vi "OP150ZP_SCANequipements.vi"(8 "Errin":errorcluster caption="errin", 10 "Chaîne":string="Log et conf\\Config.ini", 11 "pathin":path=path "D:/CODE/02 SLIM ZEN") -> (0 "ERROUT":errorcluster caption="error out", 1 "KO?":bool=TRUE)   [LabVIEW 2020]
doc: "Ce vi il détecte la presence des équipements"
uses:
  Documents/GitHub/ZEN-PLUS/OP150/EN PRODUCTION/OP150/VG/VG_BT3562.vi
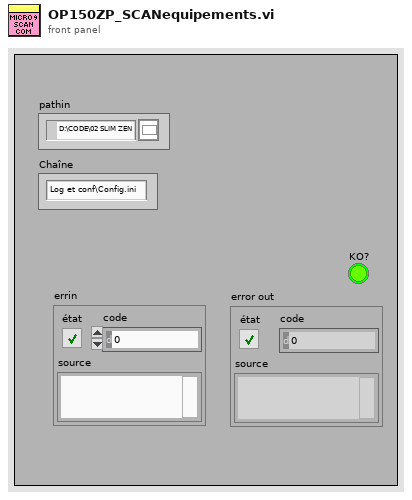
[diagram p1: front panel]
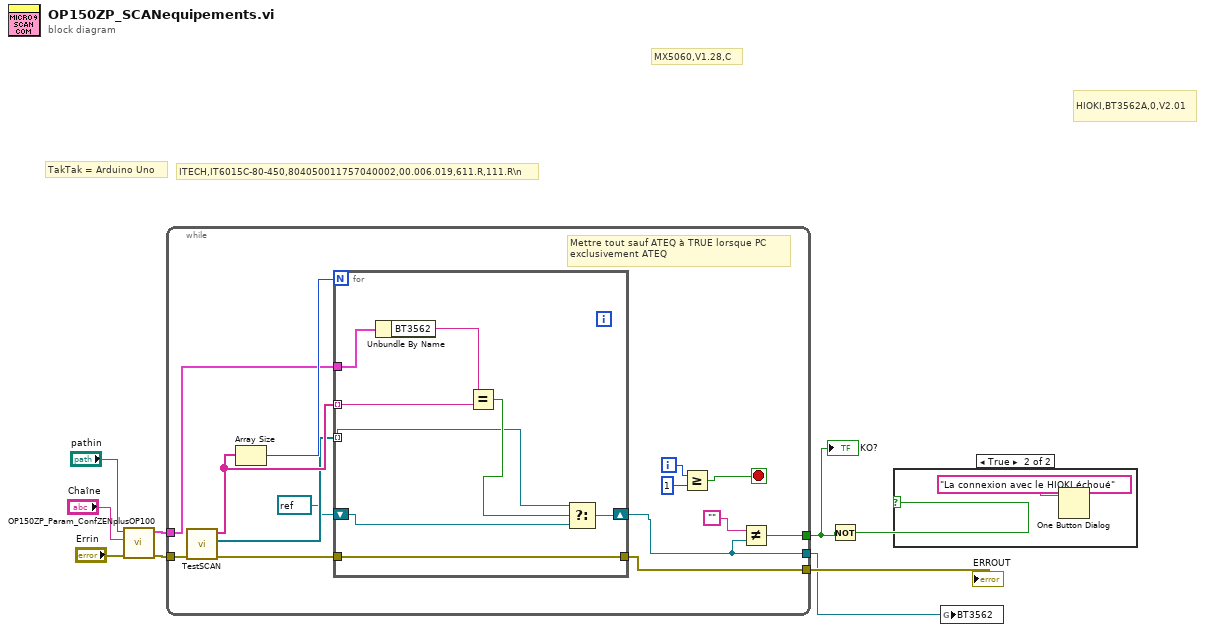
[diagram p0: block diagram]
diagram:
  # "MX5060,V1.28,C"
  # "HIOKI,BT3562A,0,V2.01"
  # "TakTak = Arduino Uno"
  # "ITECH,IT6015C-80-450,804050011757040002,00.006.019,611.R,111.R\\n"
  n1 = call "OP150ZP_Param_ConfZENplusOP100.vi"("errin"="Errin", "Chaîne"="Chaîne", "pathin"="pathin") -> ("errout"=w8:errorcluster, "VISA OUT"=w7:cluster{"BT3562":string})  [unwired: 7 in]
  n2 = while {
    tunnel: w8 -> [w22]
    tunnel: w7 -> [w17]
    tunnel: [w12] -> w3
    tunnel: [w14] -> w4
    tunnel: [w10] -> w2
    i -> [w19]
    stop <- w13 stop-if-true
    # "Mettre tout sauf ATEQ à TRUE lorsque PC \nexclusivement ATEQ"
    n3 = call <userlib>:"TestSCAN.vi"("errin"=w22) -> ("error out"=w15:errorcluster, "Tableau 2"=w20:refnum<visa-resource-name>[], "Tableau"=w21:string[])  [unwired: 8 in]
    n4 = Array Size(array=w21) -> (size(s)=w23:i32)
    n5 = for {
      N: w23 -> [_]
      tunnel: w21 -> [w28] mode=indexing
      tunnel: w17 -> [w31]
      shift-right: [w24] -> w12
      shift-left: refnum<visa-resource-name> refnum ("VISA resource name out") -> [w25]
      tunnel: w20 -> [w26] mode=indexing
      tunnel: w15 -> [w30]
      tunnel: [w30] -> w14
      n6 = Unbundle By Name(w31) -> ("BT3562"=w29:string)
      n7 = Equal?(x=w29, y=w28) -> (x = y?=w27:bool)
      n8 = Select(t=w26, s=w27, f=w25) -> (s? t:f=w24:refnum<visa-resource-name>)
    }
    n9 = Greater Or Equal?(x=w19, y=1) -> (x >= y?=w13:bool)
    n10 = Not Equal?(x="", y=w12) -> (x != y?=w10:bool)
  }
  "KO?" <- w2
  "ERROUT" <- w4
  n11 = Not(x=w2) -> (.not. x?=w1:bool)
  n12 = case shown="True" w1 {
    frame False {
    }
    frame True {
      n13 = One Button Dialog(message="La connexion avec le HIOKI échoué") -> ()  [unwired: 1 in, 1 out]
    }
  }
  n14 = global write "VG_BT3562.vi" "BT3562"(w3) -> ()
